vi "Panel.vi"(11 "Game Config Panel in":refnum<class "Game Config Panel.lvclass">) -> ()   [LabVIEW 2020, in "SB App.lvlib" / "Game Config Panel.lvclass"]
uses:
  Game Config Panel.lvclass
  C:/Program Files (x86)/National Instruments/LabVIEW 2020/vi.lib/IlluminatedG/IG OOPanel/OOPanel/Panel/Panel.lvclass
  <vilib>/IlluminatedG/IG OOPanel/OOPanel/Panel/Basic UI State.ctl
  Game Config Panel.lvclass/Game Config Panel.ctl
  <vilib>/IlluminatedG/IG OOPanel/OOPanel/ArrayManager/ArrayManager.lvclass
  Team Config Panel/Team Config Panel.lvclass
  C:/Program Files (x86)/National Instruments/LabVIEW 2020/vi.lib/IlluminatedG/IG OOPanel/OOPanel/ArrayPanel/ArrayPanel.lvclass
  SquareBattle/Team/Team.lvclass/Team.ctl
  Game Start Data.ctl
  Board Size Update.ctl
  SquareBattle/Team/Team.lvclass
  <vilib>/IlluminatedG/IG OOPanel/OOPanel/Panel/Panel.lvclass
  <vilib>/IlluminatedG/IG OOPanel/OOPanel/OOPanel.lvlib
  SquareBattle/SquareBattle.lvlib
  SB App.lvlib
  C:/dev/illuminatedg/sol-squarebattle/ProjectTemplates/Source/SummerOfLabVIEW/SquareBattle/template/SB App/Game Config Panel/Game Config Panel.lvclass
  C:/dev/illuminatedg/sol-squarebattle/ProjectTemplates/Source/SummerOfLabVIEW/SquareBattle/template/SB App/Team Config Panel/Team Config Panel.lvclass
panel:
  in  "Time Limit":i32=10
  in  "Round Limit":u32
  in  "Recording":bool
  in  "Randomize":bool
  in  "Replication Rounds":u32=50
  in  "Board Size":i32=150
  in  "Add Team":bool
  in  "Start":bool
  # "mins"
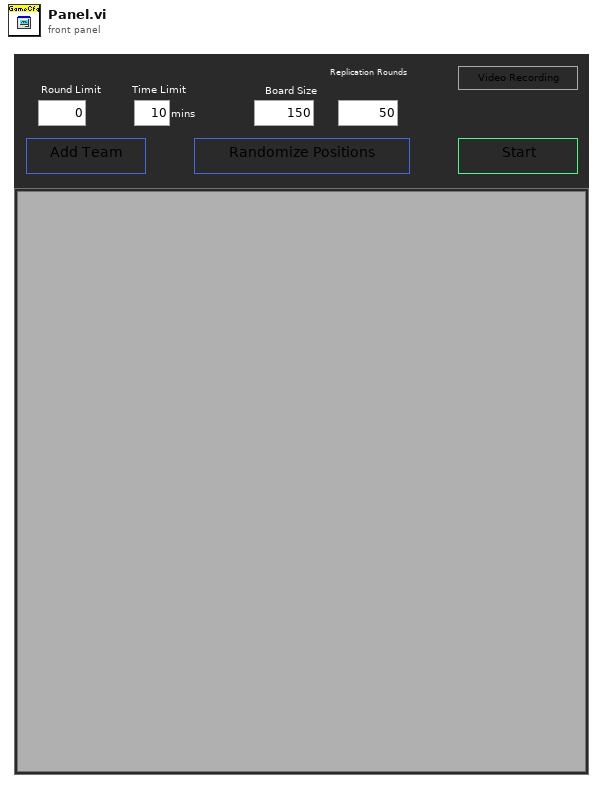
[diagram p1: front panel]
types:
  T1 = typedef "OOPanel.lvlib/Panel.lvclass/Basic UI State.ctl" = enum16{"Init", "Run", "Close"}
  T2 = enum8{"Enabled", "Disabled", "Disabled and Grayed Out"}
  T3 = typedef "SB App.lvlib/Game Start Data.ctl" = cluster{"Round Limit":u32, "Time Limit":i32}
  T4 = typedef "SB App.lvlib/Board Size Update.ctl" = cluster{"Board Size":i32}
  T5 = typedef "SB App.lvlib/Game Config Panel.lvclass/Incoming Events.ctl" = cluster{"Reset Config":refnum<user-event>, "Add Team":refnum<user-event>, "Start Position":refnum<user-event>, "Remove Team":refnum<user-event>, "Video Enabled":refnum<user-event>}
  T6 = typedef "OOPanel.lvlib/Panel.lvclass/Panel Events.ctl" = cluster{"Visbility":refnum<user-event>, "Close":refnum<user-event>}
  T7 = typedef "SquareBattle.lvlib/Team ID.ctl" = u32
  T8 = typedef "SquareBattle.lvlib/Position.ctl" = cluster{"Row":i32, "Col":i32}
  T9 = map{T7, refnum<class "Team Config Panel.lvclass">}
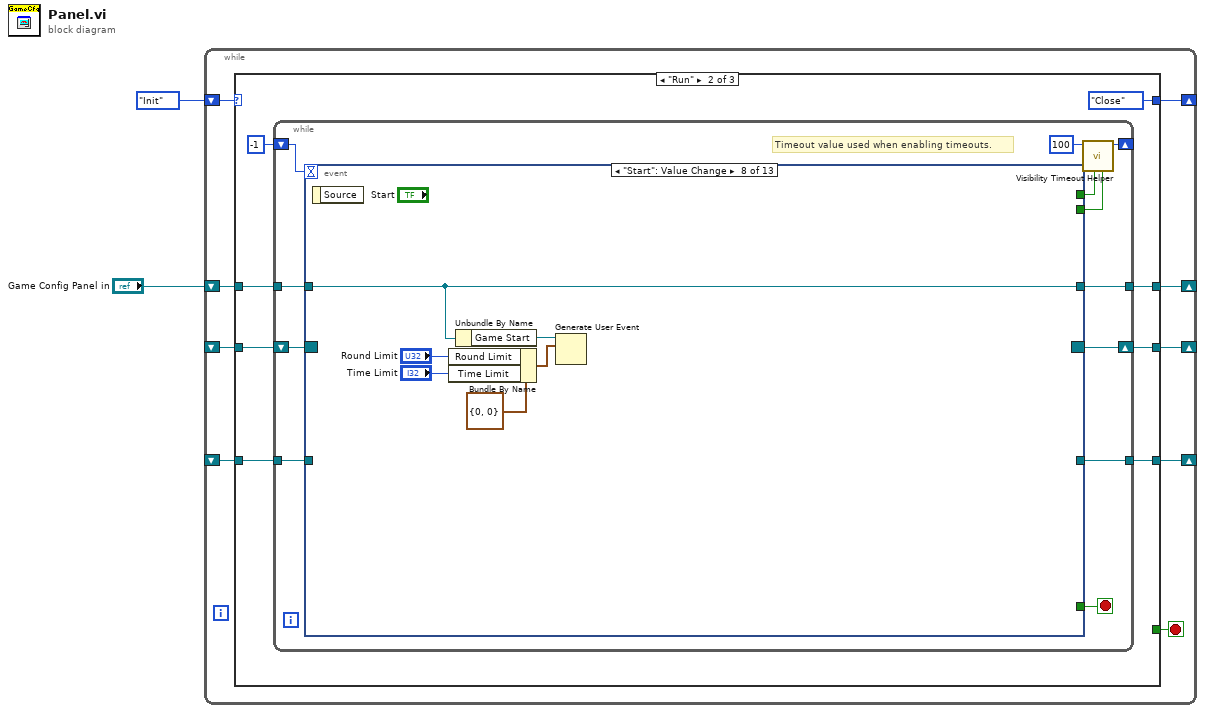
[diagram p0: block diagram]
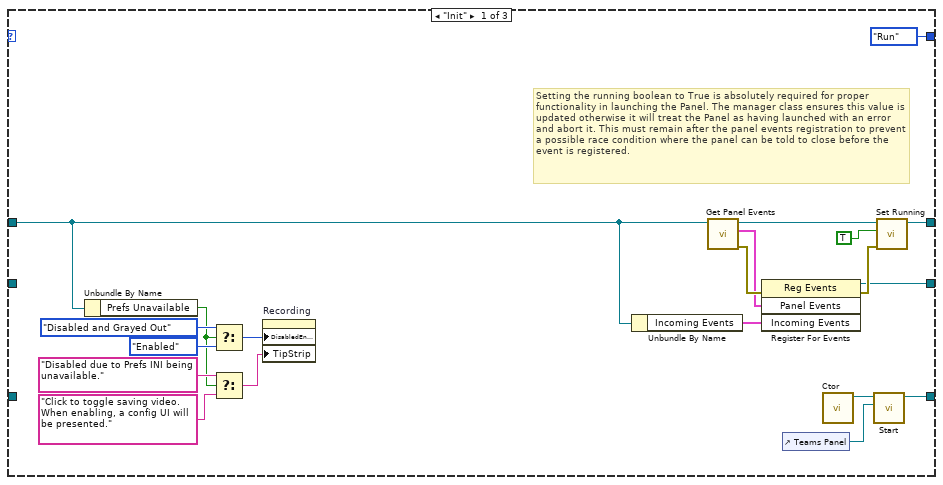
[diagram p2: hidden frame]
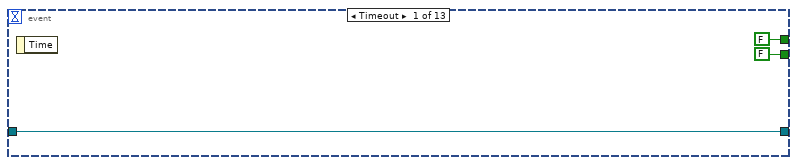
[diagram p3: hidden frame]
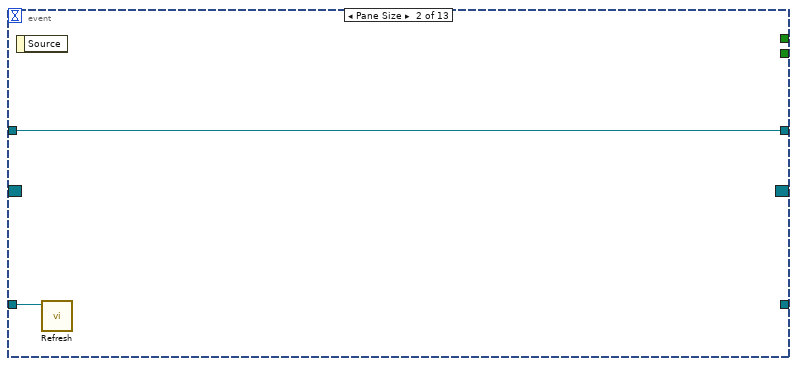
[diagram p4: hidden frame]
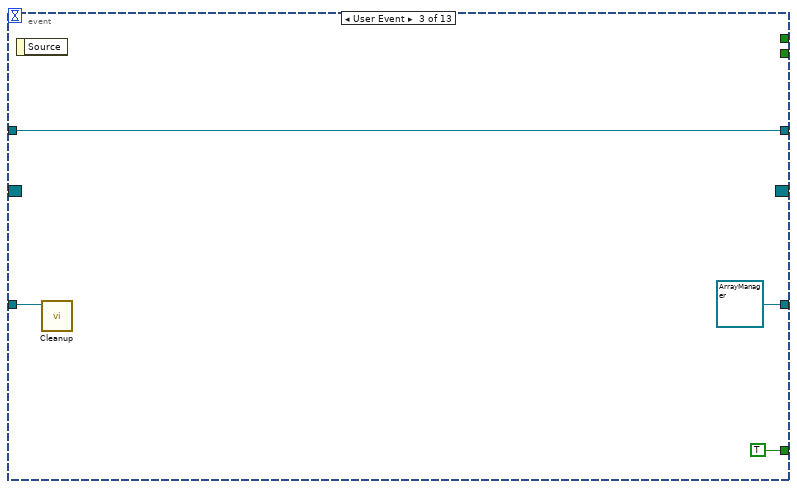
[diagram p5: hidden frame]
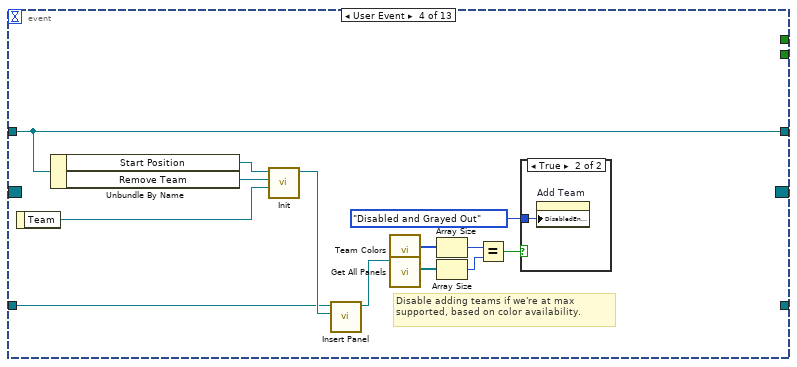
[diagram p6: hidden frame]
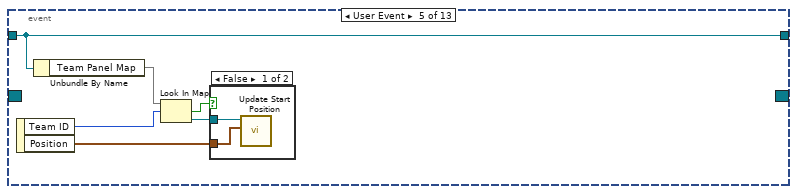
[diagram p8: hidden frame]
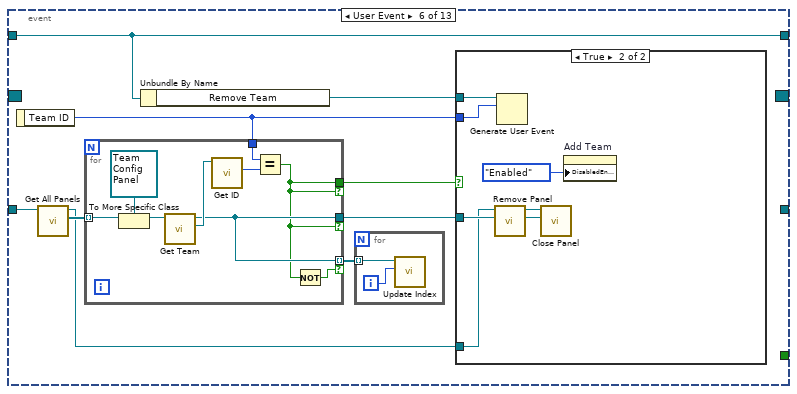
[diagram p10: hidden frame]
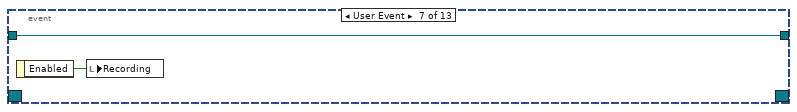
[diagram p12: hidden frame]
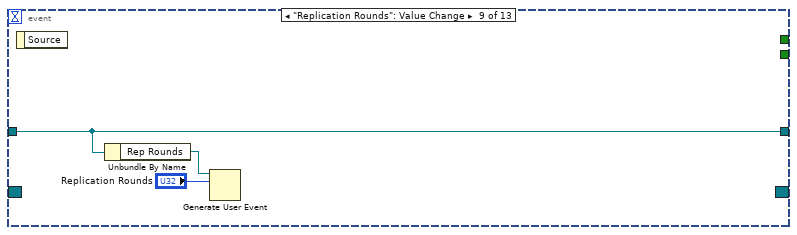
[diagram p13: hidden frame]
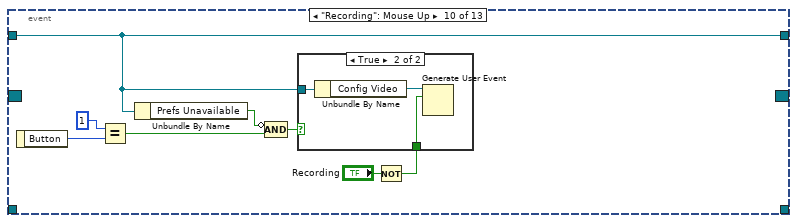
[diagram p14: hidden frame]
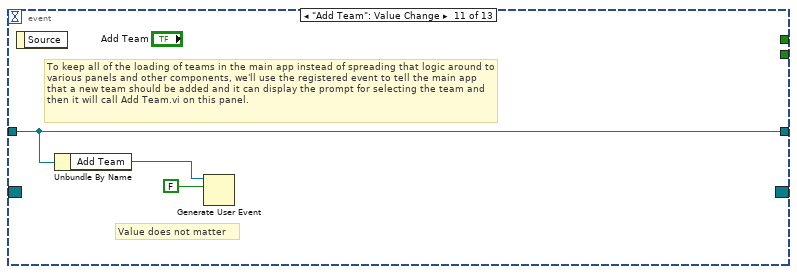
[diagram p16: hidden frame]
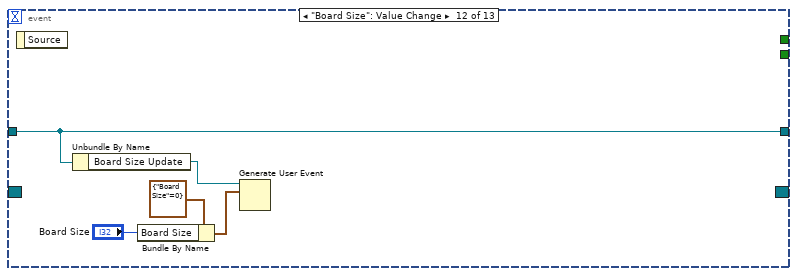
[diagram p17: hidden frame]
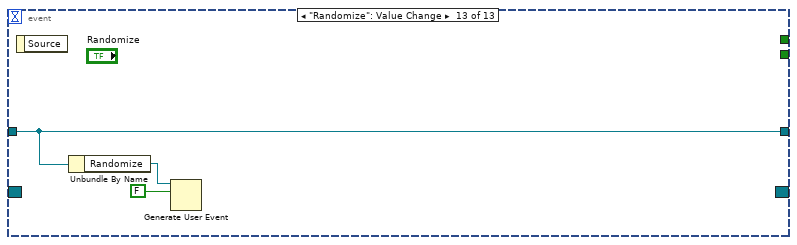
[diagram p18: hidden frame]
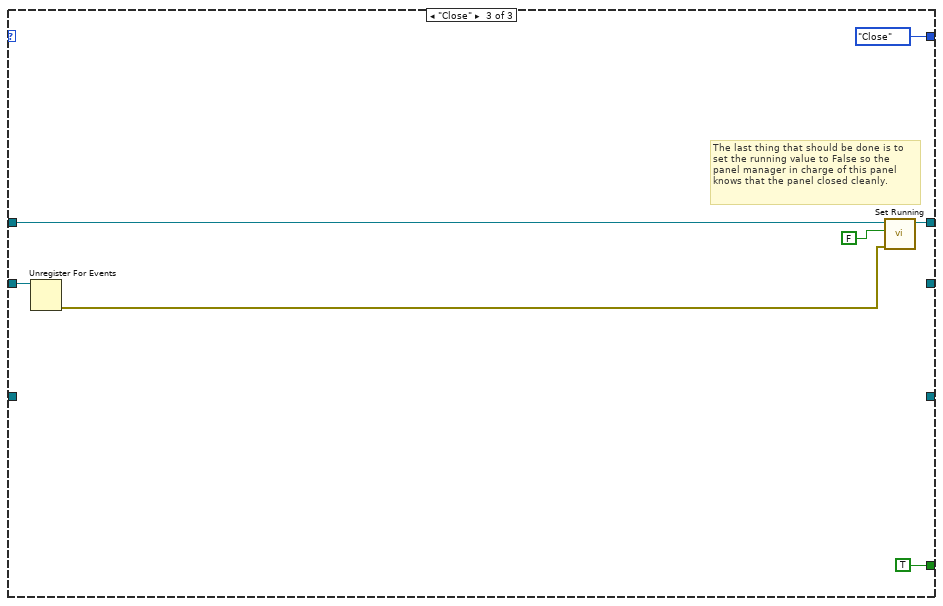
[diagram p19: hidden frame]
diagram:
  n1 = while {
    shift-right: [w10] -> _
    shift-left: _ -> [w11]
    shift-right: [w8] -> _
    shift-left: Basic_UI_State."Init" ("Basic UI State") -> [w9]
    shift-right: [w6] -> _
    shift-left: "Game Config Panel in" -> [w5]
    shift-right: [w4] -> _
    shift-left: _ -> [w3]
    stop <- w7 stop-if-true
    n2 = case shown="\"Run\"" w9 {
      tunnel: w11 -> [_ w39 w145]
      tunnel: [w25 w37 _] -> w10
      tunnel: [Basic_UI_State."Run" ("Basic UI State") Basic_UI_State."Close" ("Basic UI State") Basic_UI_State."Close" ("Basic UI State")] -> w8
      tunnel: [_ _ TRUE] -> w7
      tunnel: [w24 w34 w143] -> w6
      tunnel: w5 -> [w19 w35 w144]
      tunnel: [w20 w32 _] -> w4
      tunnel: w3 -> [_ w33 _]
      frame "Init" {
        # "Setting the running boolean to True is absolutely required for proper functionality in launching the Panel. The manager class ensures this value is updated otherwise it will treat the Panel as having launched with an error and abort it. This must remain after the panel events registration to prevent a possible race condition where the panel can be told to close before the event is registered."
        n3 = Unbundle By Name(w19) -> ("Prefs Unavailable"=w13:bool)
        n4 = Select(t=T2."Disabled and Grayed Out" ("Disabled"), s=w13, f=T2."Enabled" ("Disabled")) -> (s? t:f=w16:T2)
        n5 = Select(t="Disabled due to Prefs INI being unavailable.", s=w13, f="Click to toggle saving video. When enabling, a config UI will be presented.") -> (s? t:f=w12:string)
        n6 = property on="Recording" class="Bool (strict)"("DisabledEnum"=w16, "TipStrip"=w12) -> ()  [unwired: 2 in, 2 out]
        n7 = Unbundle By Name(w19) -> ("Incoming Events"=w23:T5)
        n8 = call <vilib>:"Get Panel Events.vi"("Panel in"=w19) -> ("error out"=w31:errorcluster, "Panel Events"=w27:T6, "Panel out"=w28:refnum<class "Game Config Panel.lvclass">)  [unwired: 8 in]
        n9 = register-events(error in=w31, w27, w23) -> (reference out=w25:refnum<event-registration>, error out=w29:errorcluster)  [unwired: 1 in]
        n10 = control-ref of="Teams Panel"() -> (w22:refnum<vi>)
        n11 = call <vilib>:"Ctor.vi"() -> ("PanelArray"=w21:refnum<class "ArrayManager.lvclass">)  [unwired: 10 in, 1 out]
        n12 = call <vilib>:"Start.vi"("Container"=w22, "ArrayManager in"=w21) -> ("ArrayManager out"=w20:refnum<class "ArrayManager.lvclass">)  [unwired: 8 in, 1 out]
        n13 = call <vilib>:"Set Running.vi"("error in (no error)"=w29, "Running"=TRUE, "Panel in"=w28) -> ("Panel out"=w24:refnum<class "Game Config Panel.lvclass">)  [unwired: 7 in, 1 out]
      }
      frame "Run" {
        n14 = while {
          shift-right: [w47] -> w37
          shift-left: w39 -> [w48]
          shift-right: [w50] -> _
          shift-left: -1 ("Timeout") -> [w49]
          tunnel: w35 -> [w43]
          tunnel: [w42] -> w34
          tunnel: w33 -> [w41]
          tunnel: [w40] -> w32
          stop <- w44 stop-if-true
          # "Timeout value used when enabling timeouts."
          n15 = event shown="[7] \"Start\": Value Change" {
            selector: w48 -> [_ _ _ _ _ _ _ _ _ _ _ _ _]
            dyn-events: [_ _ _ _ _ _ _ _ _ _ _ _ _] -> w47
            timeout: w49 -> [_ _ _ _ _ _ _ _ _ _ _ _ _]
            tunnel: [FALSE _ _ _ _ _ _ _ _ _ _ _ _] -> w46
            tunnel: [FALSE _ _ _ _ _ _ _ _ _ _ _ _] -> w45
            tunnel: [_ _ TRUE _ _ _ _ _ _ _ _ _ _] -> w44
            tunnel: w43 -> [w52 w56 w59 w73 w75 w85 w111 w117 w120 w124 w134 w139 w142]
            tunnel: [w52 w56 w59 w73 w75 w85 w111 w117 w120 w124 w134 w139 w142] -> w42
            tunnel: w41 -> [_ w55 w57 w69 _ w91 _ _ _ _ _ _ _]
            tunnel: [_ _ refnum<class "ArrayManager.lvclass"> refnum ("ArrayManager out") _ _ _ _ _ _ _ _ _ _] -> w40
            event Timeout {
              n16 = event-data() -> ()  [unwired: 1 in, 1 out]
            }
            event Pane Size {
              n17 = event-data() -> ()  [unwired: 1 in, 1 out]
              n18 = call <vilib>:"Refresh.vi"("ArrayManager in"=w55) -> ()  [unwired: 9 in, 2 out]
            }
            event User Event {
              n19 = event-data() -> ()  [unwired: 1 in, 1 out]
              n20 = call <vilib>:"Cleanup.vi"("PanelArray in"=w57) -> ()  [unwired: 10 in, 1 out]
            }
            event User Event {
              # "Disable adding teams if we're at max supported, based on color availability."
              n21 = event-data() -> ("Team"=w71:refnum<class "Team.lvclass">)  [unwired: 1 in]
              n22 = Unbundle By Name(w73) -> ("Start Position"=w70:refnum<user-event>, "Remove Team"=w61:refnum<user-event>)
              n23 = call "Init.vi"("Team"=w71, "Remove Team"=w61, "Start Position"=w70) -> ("Team Config Panel out"=w72:refnum<class "Team Config Panel.lvclass">)  [unwired: 7 in, 1 out]
              n24 = call <vilib>:"Insert Panel.vi"("Panel/Type"=w72, "PanelArray in"=w69) -> ("PanelArray out"=w68:refnum<class "ArrayManager.lvclass">)  [unwired: 7 in, 2 out]
              n25 = call "Team Colors.vi"() -> ("Team Colors"=w66:u32[])  [unwired: 11 in]
              n26 = call <vilib>:"Get All Panels.vi"("PanelArray in"=w68) -> ("Panels"=w67:refnum<class "ArrayPanel.lvclass">[])  [unwired: 8 in, 2 out]
              n27 = Array Size(array=w66) -> (size(s)=w65:i32)
              n28 = Array Size(array=w67) -> (size(s)=w64:i32)
              n29 = Equal?(x=w65, y=w64) -> (x = y?=w63:bool)
              n30 = case shown="True" w63 {
                tunnel: T2."Disabled and Grayed Out" ("Disabled") -> [_ w74]
                frame False {
                }
                frame True {
                  n31 = property on="Add Team" class="Bool"("DisabledEnum"=w74) -> ()  [unwired: 2 in, 2 out]
                }
              }
            }
            event User Event {
              n32 = event-data() -> ("Team ID"=w79:T7, "Position"=w78:T8)  [unwired: 1 in]
              n33 = Unbundle By Name(w75) -> ("Team Panel Map"=w80:T9)
              n34 = Look In Map(map=w80, key=w79) -> (key not found?=w77:bool, value=w76:refnum<class "Team Config Panel.lvclass">)  [unwired: 1 in]
              n35 = case shown="False" w77 {
                tunnel: w78 -> [w81 _]
                tunnel: w76 -> [w82 _]
                frame False {
                  n36 = call "Update Start Position.vi"("Position"=w81, "Team Config Panel in"=w82) -> ()  [unwired: 8 in, 2 out]
                }
                frame True {
                }
              }
            }
            event User Event {
              n37 = event-data() -> ("Team ID"=w86:T7)  [unwired: 1 in]
              n38 = call <vilib>:"Get All Panels.vi"("PanelArray in"=w91) -> ("Panels"=w90:refnum<class "ArrayPanel.lvclass">[], "PanelArray out"=w87:refnum<class "ArrayManager.lvclass">)  [unwired: 8 in, 1 out]
              n39 = for {
                tunnel: w90 -> [w109] mode=indexing
                tunnel: w86 -> [w104]
                tunnel: [w102] -> w89 if=w102
                tunnel: [w103] -> w88 if=w102
                tunnel: [w103] -> w83 mode=indexing if=w101
                n40 = To More Specific Class(target class=refnum<class "Team Config Panel.lvclass"> refnum ("SB App.lvlib:Team Config Panel.lvclass"), reference=w109) -> (specific class reference=w107:refnum<class "Team Config Panel.lvclass">)  [unwired: 1 in, 1 out]
                n41 = call "Get Team.vi"("Team Config Panel in"=w107) -> ("Team"=w106:refnum<class "Team.lvclass">, "Team Config Panel out"=w103:refnum<class "Team Config Panel.lvclass">)  [unwired: 8 in, 1 out]
                n42 = call "Get ID.vi"("Team in"=w106) -> ("Team ID"=w105:T7)  [unwired: 10 in]
                n43 = Equal?(x=w104, y=w105) -> (x = y?=w102:bool)
                n44 = Not(x=w102) -> (.not. x?=w101:bool)
              }
              n45 = Unbundle By Name(w85) -> ("Remove Team"=w84:refnum<user-event>)
              n46 = for {
                tunnel: w83 -> [w93] mode=indexing
                i -> [w92]
                n47 = call "Update Index.vi"("Index"=w92, "Team Config Panel in"=w93) -> ()  [unwired: 8 in, 2 out]
              }
              n48 = case shown="True" w89 {
                tunnel: w88 -> [_ w100]
                tunnel: w87 -> [_ w99]
                tunnel: w86 -> [_ w95]
                tunnel: w84 -> [_ w96]
                frame False {
                }
                frame True {
                  n49 = call <vilib>:"Remove Panel.vi"("Panel in"=w100, "ArrayManager in"=w99) -> ("Panel"=w97:refnum<class "ArrayPanel.lvclass">, "ArrayManager out"=w98:refnum<class "ArrayManager.lvclass">)  [unwired: 7 in, 1 out]
                  n50 = Generate User Event(user event=w96, event data cluster=w95) -> ()  [unwired: 2 in, 2 out]
                  n51 = call <vilib>:"Close Panel.vi"("ArrayPanel"=w97, "ArrayManager in"=w98) -> ()  [unwired: 8 in, 2 out]
                  n52 = property on="Add Team" class="Bool"("DisabledEnum"=T2."Enabled" ("Disabled")) -> ()  [unwired: 2 in, 2 out]
                }
              }
            }
            event User Event {
              n53 = event-data() -> ("Enabled"=w110:bool)  [unwired: 1 in]
              n54 = local write "Recording"(w110) -> ()
            }
            event "Start": Value Change {
              n55 = event-data() -> ()  [unwired: 1 in, 1 out]
              n56 = Bundle By Name(cluster=T3 {"Round Limit"=0, "Time Limit"=0} ("event data"), "Round Limit"="Round Limit", "Time Limit"="Time Limit") -> (w112:T3)
              n57 = Unbundle By Name(w117) -> ("Game Start"=w116:refnum<user-event>)
              n58 = Generate User Event(user event=w116, event data cluster=w112) -> ()  [unwired: 2 in, 2 out]
            }
            event "Replication Rounds": Value Change {
              n59 = event-data() -> ()  [unwired: 1 in, 1 out]
              n60 = Unbundle By Name(w120) -> ("Rep Rounds"=w119:refnum<user-event>)
              n61 = Generate User Event(user event=w119, event data cluster="Replication Rounds") -> ()  [unwired: 2 in, 2 out]
            }
            event "Recording": Mouse Up {
              n62 = event-data() -> ("Button"=w126:u16)  [unwired: 1 in]
              n63 = Equal?(x=u16 1, y=w126) -> (x = y?=w123:bool)
              n64 = Unbundle By Name(w124) -> ("Prefs Unavailable"=w122:bool)
              n65 = Compound Arithmetic op=AND(invert w122, w123) -> (w121:bool)
              n66 = Not(x="Recording") -> (.not. x?=w127:bool)
              n67 = case shown="True" w121 {
                tunnel: w124 -> [_ w131]
                tunnel: w127 -> [_ w129]
                frame False {
                }
                frame True {
                  n68 = Unbundle By Name(w131) -> ("Config Video"=w130:refnum<user-event>)
                  n69 = Generate User Event(user event=w130, event data cluster=w129) -> ()  [unwired: 2 in, 2 out]
                }
              }
            }
            event "Add Team": Value Change {
              # "Value does not matter"
              # "To keep all of the loading of teams in the main app instead of spreading that logic around to various panels and other components, we'll use the registered event to tell the main app that a new team should be added and it can display the prompt for selecting the team and then it will call Add Team.vi on this panel."
              n70 = event-data() -> ()  [unwired: 1 in, 1 out]
              n71 = Unbundle By Name(w134) -> ("Add Team"=w133:refnum<user-event>)
              n72 = Generate User Event(user event=w133, event data cluster=FALSE ("event data")) -> ()  [unwired: 2 in, 2 out]
            }
            event "Board Size": Value Change {
              n73 = event-data() -> ()  [unwired: 1 in, 1 out]
              n74 = Unbundle By Name(w139) -> ("Board Size Update"=w138:refnum<user-event>)
              n75 = Bundle By Name(cluster=T4 {"Board Size"=0} ("event data"), "Board Size"="Board Size") -> (w136:T4)
              n76 = Generate User Event(user event=w138, event data cluster=w136) -> ()  [unwired: 2 in, 2 out]
            }
            event "Randomize": Value Change {
              n77 = event-data() -> ()  [unwired: 1 in, 1 out]
              n78 = Unbundle By Name(w142) -> ("Randomize"=w141:refnum<user-event>)
              n79 = Generate User Event(user event=w141, event data cluster=FALSE ("event data")) -> ()  [unwired: 2 in, 2 out]
            }
          }
          n80 = call <vilib>:"Visibility Timeout Helper.vi"("Update?"=w45, "Use Timeout?"=w46, "Visible Timeout mS"=100) -> ("Timeout"=w50:i32)  [unwired: 8 in]
        }
      }
      frame "Close" {
        # "The last thing that should be done is to set the running value to False so the panel manager in charge of this panel knows that the panel closed cleanly."
        n81 = Unregister For Events(event registration refnum=w145) -> (error out=w147:errorcluster)  [unwired: 1 in]
        n82 = call <vilib>:"Set Running.vi"("error in (no error)"=w147, "Running"=FALSE, "Panel in"=w144) -> ("Panel out"=w143:refnum<class "Game Config Panel.lvclass">)  [unwired: 7 in, 1 out]
      }
    }
  }
